vi "EscapeForVarIDURL.vi"(5 "Unescaped String":string) -> (2 "VarID URL String":string)   [LabVIEW 2013]
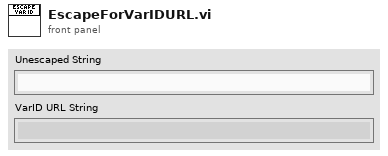
[diagram p1: front panel]
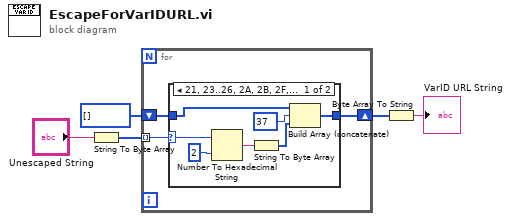
[diagram p0: block diagram]
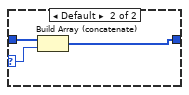
[diagram p2: hidden frame]
diagram:
  n1 = String To Byte Array(string="Unescaped String") -> (unsigned byte array=w4:u8[])
  n2 = for {
    tunnel: w4 -> [w8] mode=indexing
    shift-right: [w6] -> w1
    shift-left: u8[] [] ("unsigned byte array") -> [w7]
    n3 = case shown="21, 23..26, 2A, 2B, 2F, 3A, 3B, 3D, 3F, 40, 5B, 5D" w8 {
      selector: w8 -> [w12 w17]
      tunnel: w7 -> [w15 w18]
      tunnel: [w14 w16] -> w6
      frame 33, 35..38, 42, 43, 47, 58, 59, 61, 63, 64, 91, 93 {
        n4 = Number To Hexadecimal String(1:i16 2 ("width (-)"), 2:w12) -> (0:w10:string)
        n5 = String To Byte Array(string=w10) -> (unsigned byte array=w9:u8[])
        n6 = Build Array (concatenate)(w15, u8 37, w9) -> (w14:u8[])
      }
      frame Default {
        n7 = Build Array (concatenate)(w18, w17) -> (w16:u8[])
      }
    }
  }
  n8 = Byte Array To String(unsigned byte array=w1) -> (string=→"VarID URL String":string)
